vi "Table_AssertColumnValue_Tests.vi"(8 "error in":errorcluster) -> (0 "error out":errorcluster)   [LabVIEW 2016, in "DronaTest.lvlib"]
uses:
  DronaTest.lvlib
  APIs/Stimulus/ControlValue/SetValueAuto.vi
  APIs/Assert/AssertControlValue/Controls/Table/AssertColumnValue.vi
  <vilib>/addons/_JKI Toolkits/Caraya/classes/Assert/Assert Equal Value_Variant.vi
  <vilib>/addons/_JKI Toolkits/Caraya/classes/Test/Test.lvclass
  <vilib>/SLL Toolkit/SLL Debug/SLL Debug.lvlib
  Drona.lvlib
  <vilib>/addons/_JKI Toolkits/Caraya/classes/Assert/Assert.lvclass
  APIs/Get/GetControlRef/GetControlRef.lvlib
  APIs/Assert/AssertControlValue/Controls/Table/AssertTable.lvlib
  APIs/Stimulus/ControlValue/ControlValue.lvlib
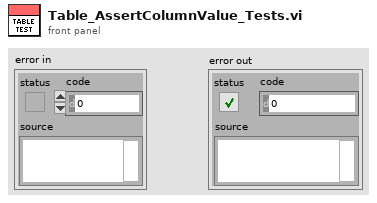
[diagram p1: front panel]
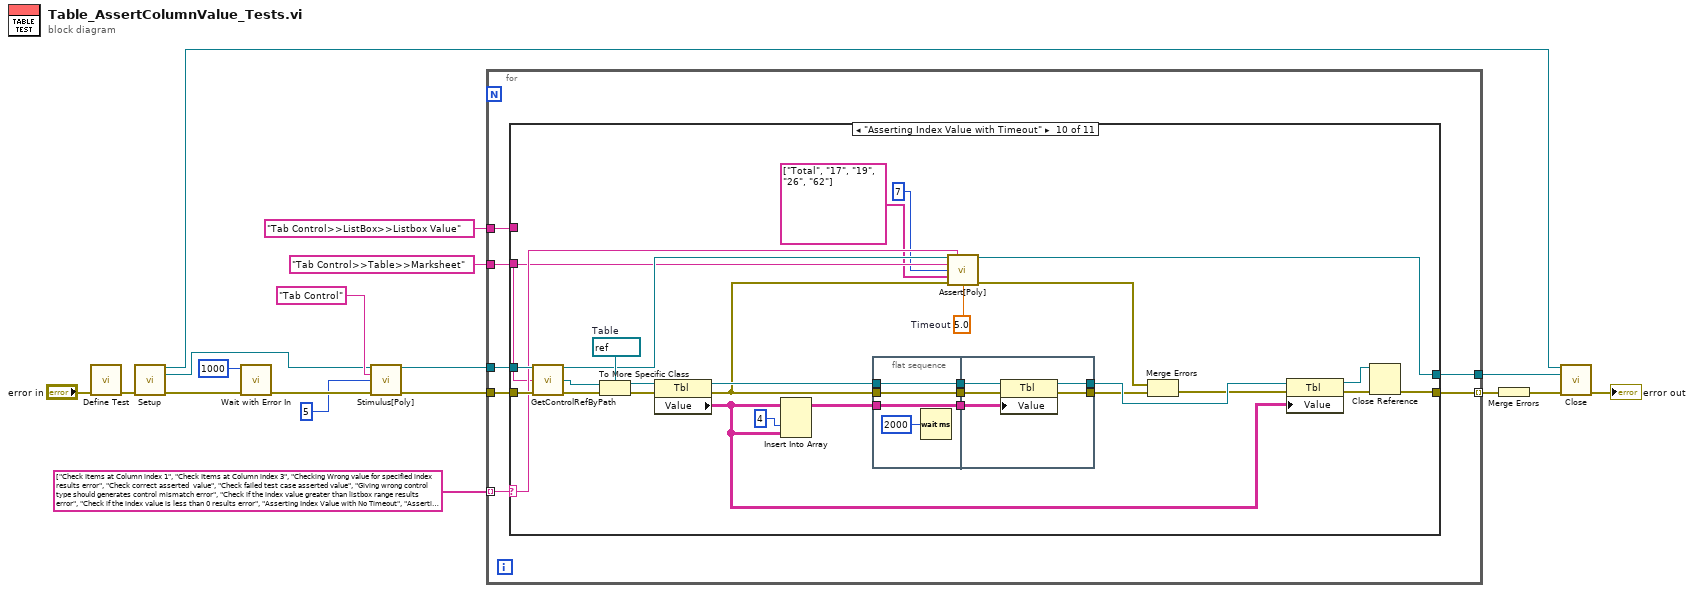
[diagram p0: block diagram]
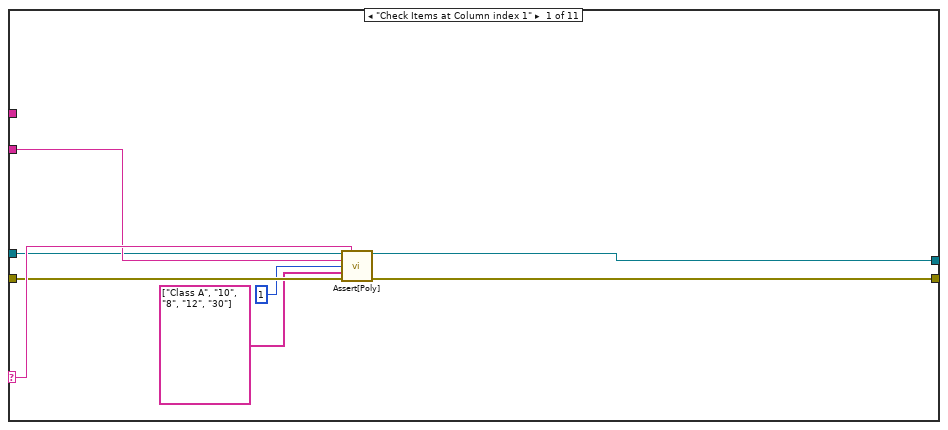
[diagram p2: hidden frame]
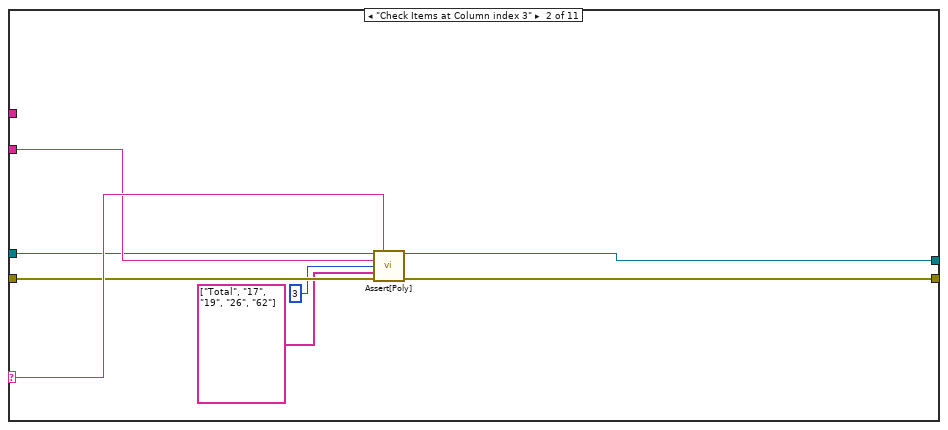
[diagram p3: hidden frame]
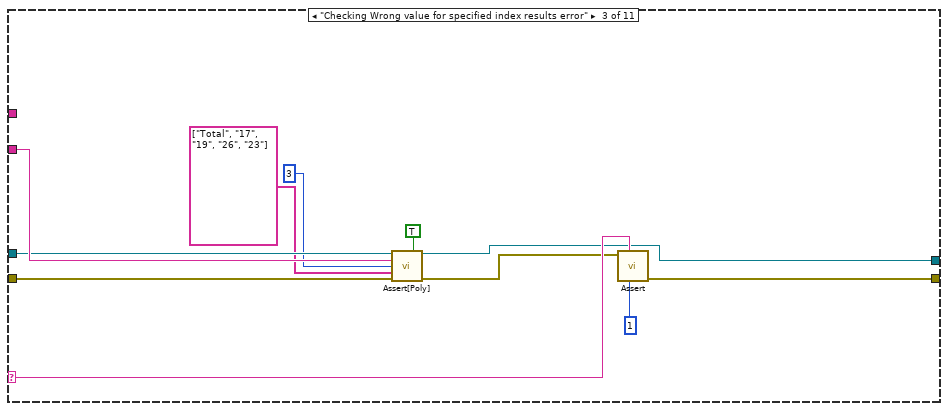
[diagram p4: hidden frame]
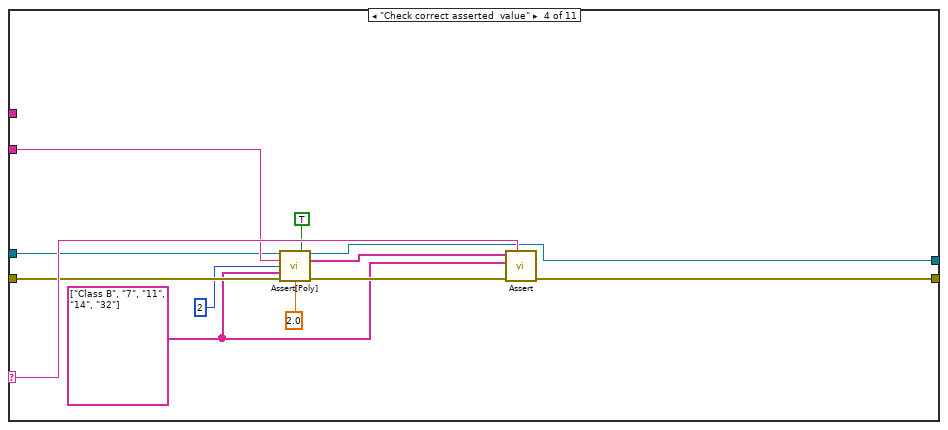
[diagram p5: hidden frame]
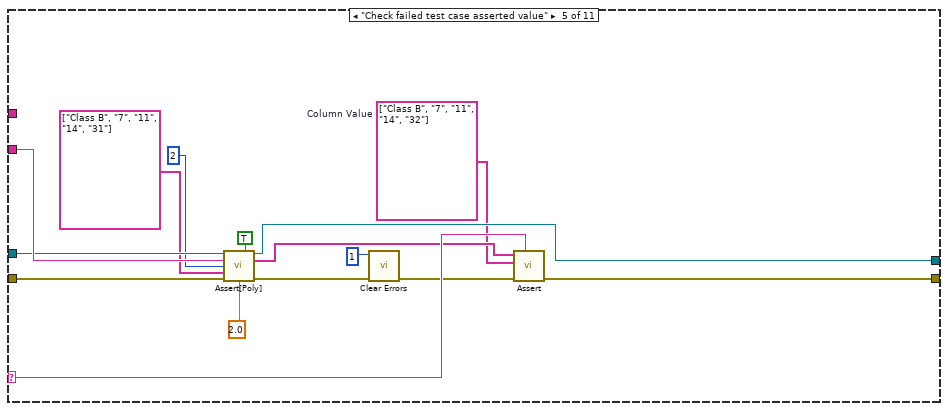
[diagram p6: hidden frame]
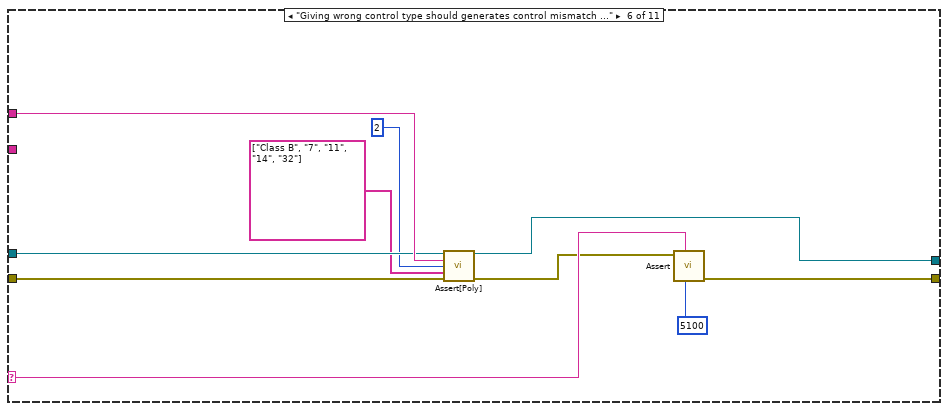
[diagram p7: hidden frame]
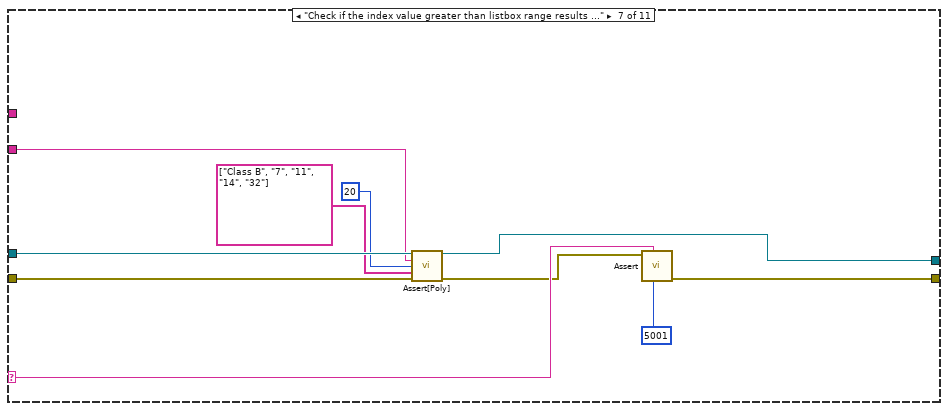
[diagram p8: hidden frame]
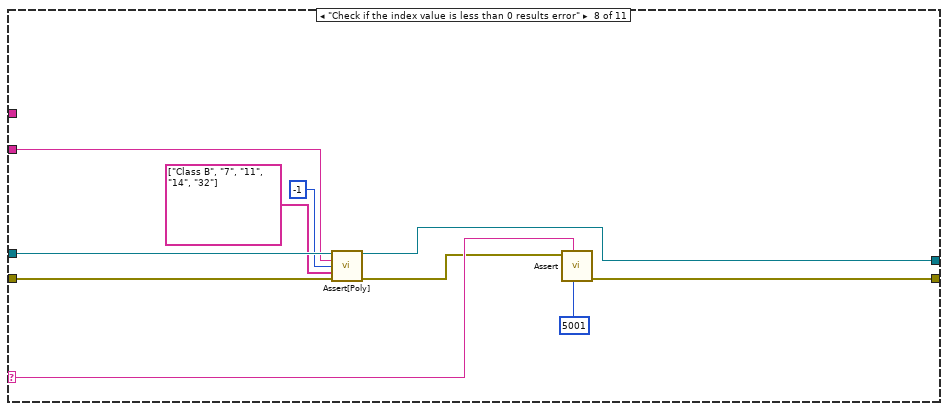
[diagram p9: hidden frame]
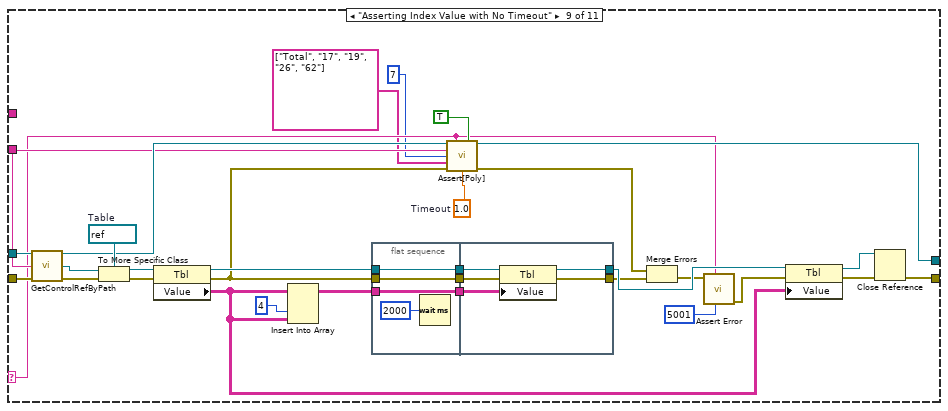
[diagram p10: hidden frame]
diagram:
  n1 = call <vilib>:"Define Test.vi"("error in (no error)"="error in") -> ("error out"=w7:errorcluster)  [unwired: 9 in, 1 out]
  n2 = call "Setup.vi"("error in"=w7) -> ("Application Ref"=w3:refnum<vi>, "VI Reference Out"=w5:refnum<vi>, "error out"=w6:errorcluster)  [unwired: 12 in]
  n3 = call <vilib>:"Wait with Error In.vi"("error in (no error)"=w6, "milliseconds to wait"=u32 1000) -> ("error out"=w16:errorcluster)  [unwired: 9 in]
  n4 = call-poly "Stimulus[Poly].vi"("VI Reference In"=w5, "Control Path"="Tab Control", "Value (Signaling)"=5, "error in"=w16) -> ("VI Reference Out"=w12:refnum<vi>, "error out"=w15:errorcluster)  [unwired: 10 in]
  n5 = for {
    tunnel: w12 -> [w21]
    tunnel: "Tab Control>>Table>>Marksheet" ("Control Path") -> [w19]
    tunnel: "Tab Control>>ListBox>>Listbox Value" ("Control Path") -> [w20]
    tunnel: string[] ["Check Items at Column index 1", "Check Items at Column index 3", "Checking Wrong value for specified index results error", "Check correct asserted  value", "Check failed test case asserted value", "Giving wrong control type should generates control mismatch error", "Check if the index value greater than listbox range results error", "Check if the index value is less than 0 results error", "Asserting Index Value with No Timeout", "Asserting Index Value with Timeout"] -> [w25] mode=indexing
    tunnel: [w23] -> w2
    tunnel: w15 -> [w22]
    tunnel: [w24] -> w8 mode=indexing
    n6 = case shown="\"Asserting Index Value with Timeout\"" w25 {
      selector: w25 -> [w31 w39 w51 w63 w78 w88 w98 w108 w115 w169 _]
      tunnel: w22 -> [w29 w37 w45 w59 w74 w83 w94 w104 w141 w179 w190]
      tunnel: w21 -> [w28 w36 w44 w58 w73 w82 w93 w103 w139 w177 w189]
      tunnel: w19 -> [w30 w38 w49 w62 w77 _ w92 w102 w131 w168 _]
      tunnel: w20 -> [_ _ _ _ _ w85 _ _ _ _ _]
      tunnel: [w33 w41 w52 w64 w79 w89 w99 w109 w127 w164 w190] -> w24
      tunnel: [w32 w40 w48 w61 w76 w84 w95 w105 w132 w170 w189] -> w23
      frame "Check Items at Column index 1" {
        n7 = call-poly "Assert[Poly].vi"("VI Reference In"=w28, "Test Label"=w31, "Control Path"=w30, "Column Index"=1 ("Item Index"), "Item Value"=string[] ["Class A", "10", "8", "12", "30"] ("Column Value"), "Error In"=w29) -> ("VI Reference Out"=w32:refnum<vi>, "Error Out"=w33:errorcluster)  [unwired: 7 in, 1 out]
      }
      frame "Check Items at Column index 3" {
        n8 = call-poly "Assert[Poly].vi"("VI Reference In"=w36, "Test Label"=w39, "Control Path"=w38, "Column Index"=3 ("Item Index"), "Item Value"=string[] ["Total", "17", "19", "26", "62"] ("Column Value"), "Error In"=w37) -> ("VI Reference Out"=w40:refnum<vi>, "Error Out"=w41:errorcluster)  [unwired: 7 in, 1 out]
      }
      frame "Checking Wrong value for specified index results error" {
        n9 = call-poly "Assert[Poly].vi"("VI Reference In"=w44, "Assert Only? (F)"=TRUE, "Control Path"=w49, "Column Index"=3 ("Item Index"), "Item Value"=string[] ["Total", "17", "19", "26", "23"] ("Column Value"), "Error In"=w45) -> ("VI Reference Out"=w48:refnum<vi>, "Error Out"=w47:errorcluster)  [unwired: 7 in, 1 out]
        n10 = call-poly <vilib>:"Assert.vi"("error code (1)"=1, "Label"=w51, "Error?"=w47) -> ("error out"=w52:errorcluster)  [unwired: 7 in, 1 out]
      }
      frame "Check correct asserted  value" {
        w53 = string[] ["Class B", "7", "11", "14", "32"] ("Column Value")
        n11 = call-poly "Assert[Poly].vi"("VI Reference In"=w58, "Assert Only? (F)"=TRUE, "Control Path"=w62, "Column Index"=2 ("Item Index"), "Item Value"=w53, "Error In"=w59, "Timeout(5 sec)"=2.0) -> ("VI Reference Out"=w61:refnum<vi>, "Asserted Value"=w56:string[], "Error Out"=w57:errorcluster)  [unwired: 6 in]
        n12 = call-poly <vilib>:"Assert.vi"("Label"=w63, "error in (no error)"=w57, "Y"=w53, "X"=w56) -> ("error out"=w64:errorcluster)  [unwired: 6 in, 1 out]
      }
      frame "Check failed test case asserted value" {
        w65 = string[] ["Class B", "7", "11", "14", "32"]  # Column Value
        n13 = call-poly "Assert[Poly].vi"("VI Reference In"=w73, "Assert Only? (F)"=TRUE, "Control Path"=w77, "Column Index"=2 ("Item Index"), "Item Value"=string[] ["Class B", "7", "11", "14", "31"] ("Column Value"), "Error In"=w74, "Timeout(5 sec)"=2.0) -> ("VI Reference Out"=w76:refnum<vi>, "Asserted Value"=w71:string[], "Error Out"=w72:errorcluster)  [unwired: 6 in]
        n14 = call <vilib>:"Clear Errors.vi"("error in (no error)"=w72, "specific error code to clear (0: all)"=1) -> ("error out"=w70:errorcluster)  [unwired: 4 in, 1 out]
        n15 = call-poly <vilib>:"Assert.vi"("Label"=w78, "error in (no error)"=w70, "Y"=w65, "X"=w71) -> ("error out"=w79:errorcluster)  [unwired: 6 in, 1 out]
      }
      frame "Giving wrong control type should generates control mismatch error" {
        n16 = call-poly "Assert[Poly].vi"("VI Reference In"=w82, "Control Path"=w85, "Column Index"=2 ("Item Index"), "Item Value"=string[] ["Class B", "7", "11", "14", "32"] ("Column Value"), "Error In"=w83) -> ("VI Reference Out"=w84:refnum<vi>, "Error Out"=w86:errorcluster)  [unwired: 8 in, 1 out]
        n17 = call-poly <vilib>:"Assert.vi"("error code (1)"=5100, "Label"=w88, "Error?"=w86) -> ("error out"=w89:errorcluster)  [unwired: 7 in, 1 out]
      }
      frame "Check if the index value greater than listbox range results error" {
        n18 = call-poly "Assert[Poly].vi"("VI Reference In"=w93, "Control Path"=w92, "Column Index"=20 ("Item Index"), "Item Value"=string[] ["Class B", "7", "11", "14", "32"] ("Column Value"), "Error In"=w94) -> ("VI Reference Out"=w95:refnum<vi>, "Error Out"=w96:errorcluster)  [unwired: 8 in, 1 out]
        n19 = call-poly <vilib>:"Assert.vi"("error code (1)"=5001, "Label"=w98, "Error?"=w96) -> ("error out"=w99:errorcluster)  [unwired: 7 in, 1 out]
      }
      frame "Check if the index value is less than 0 results error" {
        n20 = call-poly "Assert[Poly].vi"("VI Reference In"=w103, "Control Path"=w102, "Column Index"=-1 ("Item Index"), "Item Value"=string[] ["Class B", "7", "11", "14", "32"] ("Column Value"), "Error In"=w104) -> ("VI Reference Out"=w105:refnum<vi>, "Error Out"=w106:errorcluster)  [unwired: 8 in, 1 out]
        n21 = call-poly <vilib>:"Assert.vi"("error code (1)"=5001, "Label"=w108, "Error?"=w106) -> ("error out"=w109:errorcluster)  [unwired: 7 in, 1 out]
      }
      frame "Asserting Index Value with No Timeout" {
        w124 = 1.0  # Timeout
        w136 = refnum<vi> refnum  # Table
        n22 = call "GetControlRefByPath.vi"("VI Reference In"=w139, "Control Path"=w131, "error In"=w141) -> ("VI Reference Out"=w133:refnum<vi>, "Ctl Refnum"=w137:refnum<vi>, "error out"=w140:errorcluster)  [unwired: 10 in]
        n23 = To More Specific Class(target class=w136, reference=w137, error in=w140) -> (specific class reference=w135:refnum<vi>, error out=w138:errorcluster)
        n24 = property class="Tbl"(reference=w135, error in=w138) -> (reference out=w130:refnum<vi>, error out=w123:errorcluster, "Value"=w111:string[][])
        n25 = Insert Into Array(array=w111, index (col)=4 ("disabled index (col)"), new element=w111) -> (w134:string[][])  [unwired: 1 in]
        n26 = flat-sequence {
          tunnel: w123 -> [w143]
          tunnel: w130 -> [w144]
          tunnel: w134 -> [w145]
          tunnel: [w145] -> w121
          tunnel: [w144] -> w120
          tunnel: [w143] -> w119
          tunnel: [w148] -> w126
          tunnel: [w146] -> w122
          tunnel: w121 -> [w150]
          tunnel: w120 -> [w149]
          tunnel: w119 -> [w147]
          frame #0 {
            n27 = Wait (ms)(milliseconds to wait=u32 2000) -> ()  [unwired: 1 out]
          }
          frame #1 {
            n28 = property class="Tbl"(reference=w149, error in=w147, "Value"=w150) -> (reference out=w148:refnum<vi>, error out=w146:errorcluster)
          }
        }
        n29 = call-poly "Assert[Poly].vi"("VI Reference In"=w133, "Test Label"=w115, "Assert Only? (F)"=TRUE, "Control Path"=w131, "Column Index"=7 ("Row Index"), "Item Value"=string[] ["Total", "17", "19", "26", "62"] ("Column Value"), "Error In"=w123, "Timeout(5 sec)"=w124) -> ("VI Reference Out"=w132:refnum<vi>, "Error Out"=w129:errorcluster)  [unwired: 5 in, 1 out]
        n30 = Merge Errors(w129, w122) -> (w118:errorcluster)
        n31 = call <vilib>:"Assert Error.vi"("error code (1)"=5001, "Label"=w115, "Error?"=w118) -> ("error out"=w117:errorcluster)  [unwired: 7 in, 1 out]
        n32 = property class="Tbl"(reference=w126, error in=w117, "Value"=w111) -> (reference out=w125:refnum<vi>, error out=w128:errorcluster)
        n33 = Close Reference(reference=w125, error in (no error)=w128) -> (error out=w127:errorcluster)
      }
      frame "Asserting Index Value with Timeout" {
        w155 = 5.0  # Timeout
        w174 = refnum<vi> refnum  # Table
        n34 = call "GetControlRefByPath.vi"("VI Reference In"=w177, "Control Path"=w168, "error In"=w179) -> ("VI Reference Out"=w171:refnum<vi>, "Ctl Refnum"=w175:refnum<vi>, "error out"=w178:errorcluster)  [unwired: 10 in]
        n35 = To More Specific Class(target class=w174, reference=w175, error in=w178) -> (specific class reference=w173:refnum<vi>, error out=w176:errorcluster)
        n36 = property class="Tbl"(reference=w173, error in=w176) -> (reference out=w167:refnum<vi>, error out=w161:errorcluster, "Value"=w154:string[][])
        n37 = Insert Into Array(array=w154, index (col)=4 ("disabled index (col)"), new element=w154) -> (w172:string[][])  [unwired: 1 in]
        n38 = flat-sequence {
          tunnel: w161 -> [w181]
          tunnel: w167 -> [w182]
          tunnel: w172 -> [w183]
          tunnel: [w183] -> w158
          tunnel: [w182] -> w157
          tunnel: [w181] -> w156
          tunnel: [w186] -> w163
          tunnel: [w184] -> w159
          tunnel: w158 -> [w188]
          tunnel: w157 -> [w187]
          tunnel: w156 -> [w185]
          frame #0 {
            n39 = Wait (ms)(milliseconds to wait=u32 2000) -> ()  [unwired: 1 out]
          }
          frame #1 {
            n40 = property class="Tbl"(reference=w187, error in=w185, "Value"=w188) -> (reference out=w186:refnum<vi>, error out=w184:errorcluster)
          }
        }
        n41 = call-poly "Assert[Poly].vi"("VI Reference In"=w171, "Test Label"=w169, "Control Path"=w168, "Column Index"=7 ("Row Index"), "Item Value"=string[] ["Total", "17", "19", "26", "62"] ("Column Value"), "Error In"=w161, "Timeout(5 sec)"=w155) -> ("VI Reference Out"=w170:refnum<vi>, "Error Out"=w166:errorcluster)  [unwired: 6 in, 1 out]
        n42 = Merge Errors(w166, w159) -> (w160:errorcluster)
        n43 = property class="Tbl"(reference=w163, error in=w160, "Value"=w154) -> (reference out=w162:refnum<vi>, error out=w165:errorcluster)
        n44 = Close Reference(reference=w162, error in (no error)=w165) -> (error out=w164:errorcluster)
      }
      frame Default {
      }
    }
  }
  n45 = Merge Errors(w8) -> (w4:errorcluster)
  n46 = call "Close.vi"("Application Ref"=w3, "VI Reference"=w2, "error in"=w4) -> ("error out"=→"error out":errorcluster)  [unwired: 12 in]
